vi "StopTempSweep.vi"() -> ()   [LabVIEW 2013]
panel:
  in  "Stop Temp":bool
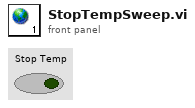
[diagram p1: front panel]
diagram:
